vi "Main.vi"(8 "error in":errorcluster, 11 "Caméra UI in":refnum<class "Caméra UI.lvclass">) -> (0 "error out":errorcluster, 3 "Caméra UI out":refnum<class "Caméra UI.lvclass">)   [LabVIEW 2026, in "Caméra UI.lvclass"]
doc: "The <b>Queued Message Handler</b> of the Worker that owns this VI."
uses:
  C:/Program Files/National Instruments/LabVIEW 2026/vi.lib/addons/_Workers/Library/Classes/Worker/Worker.lvclass
  Initialization Data.ctl
  Response Cases.ctl
  <vilib>/addons/_Workers/Library/Classes/Message Queue/Message Queue.lvclass
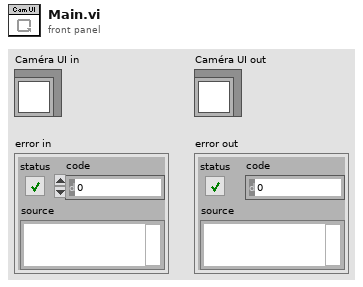
[diagram p1: front panel]
types:
  T1 = typedef "Caméra UI.lvclass/Initialization Data.ctl" = cluster{"Response Cases":T2}
  T2 = typedef "Caméra UI.lvclass/Response Cases.ctl" = cluster{"Placeholder - Can be deleted":string}
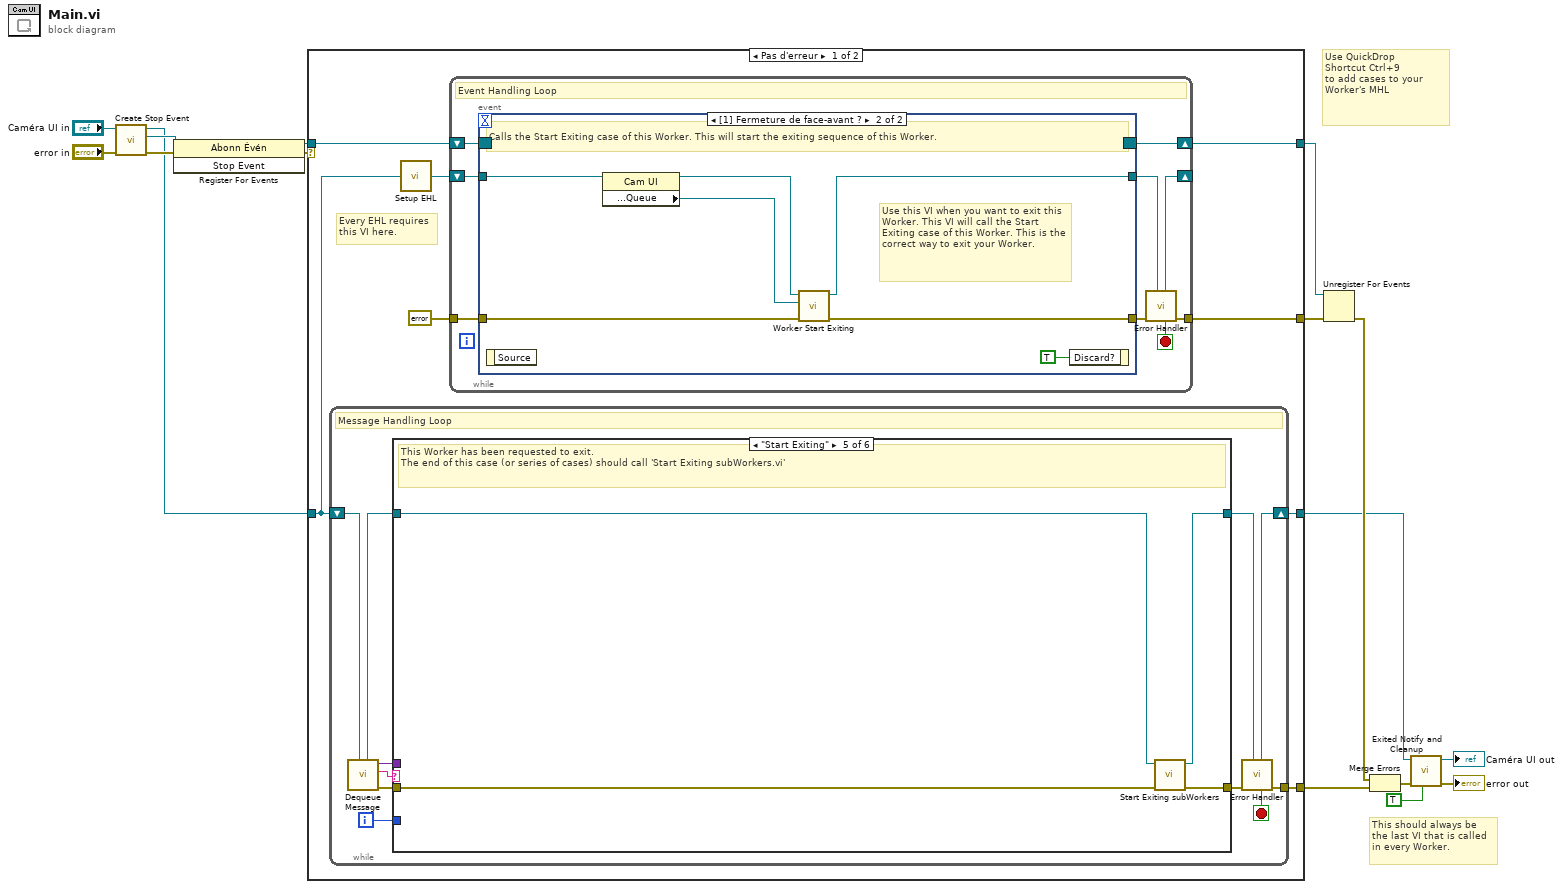
[diagram p0: block diagram]
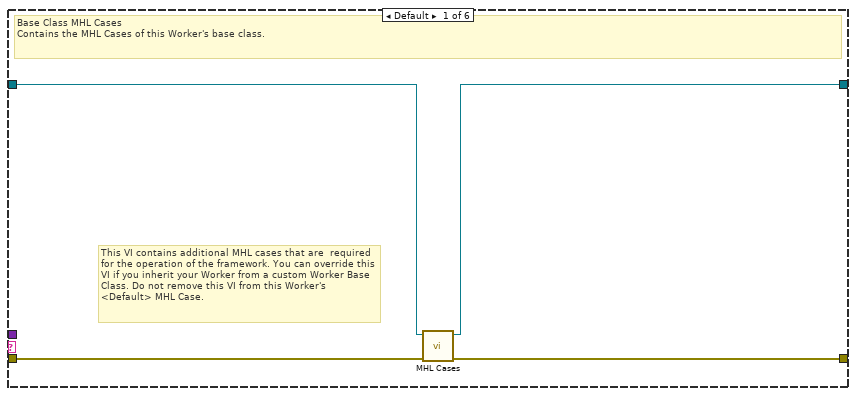
[diagram p2: hidden frame]
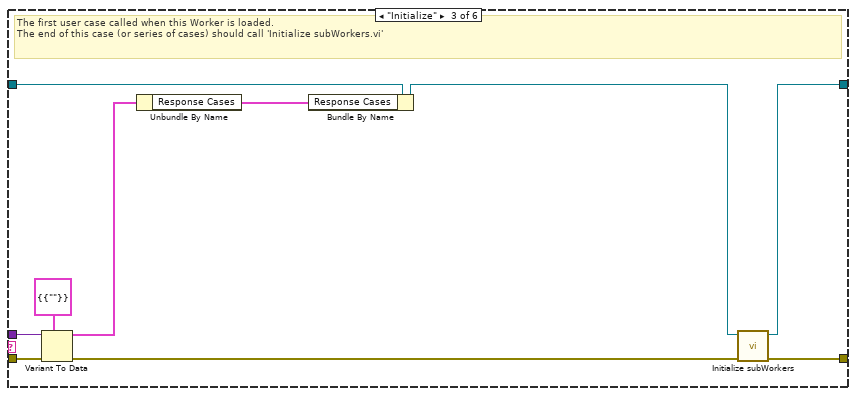
[diagram p4: hidden frame]
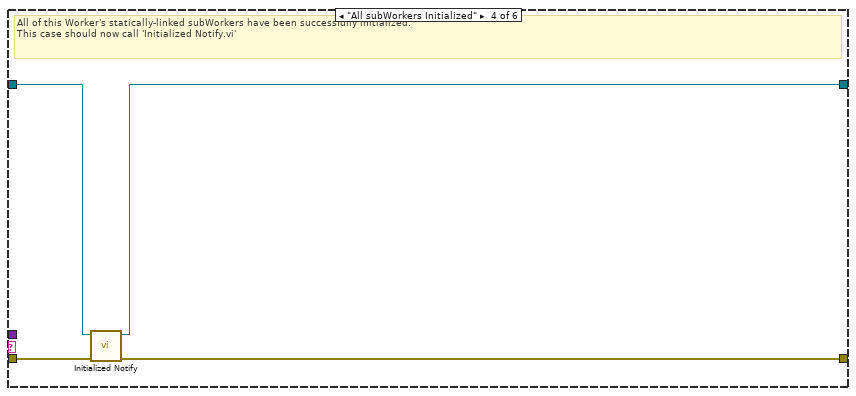
[diagram p5: hidden frame]
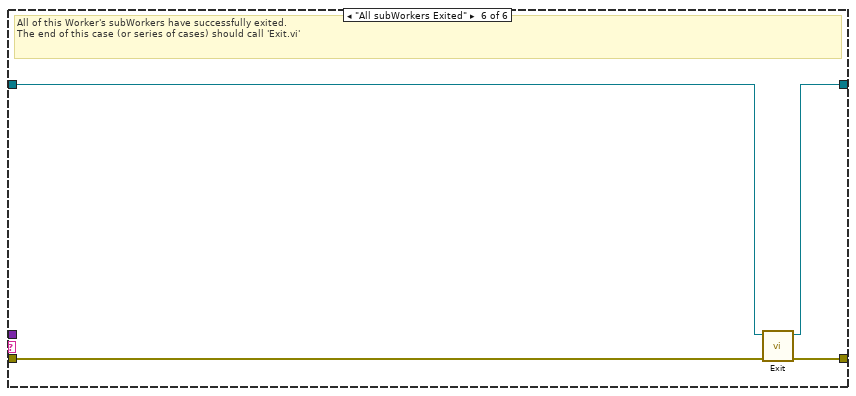
[diagram p6: hidden frame]
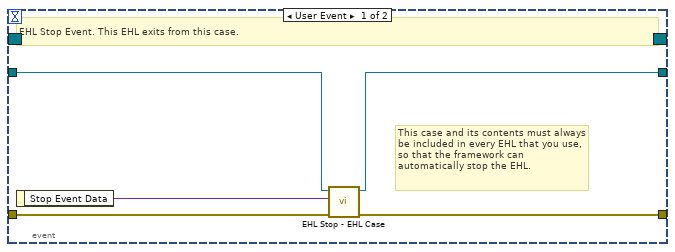
[diagram p7: hidden frame]
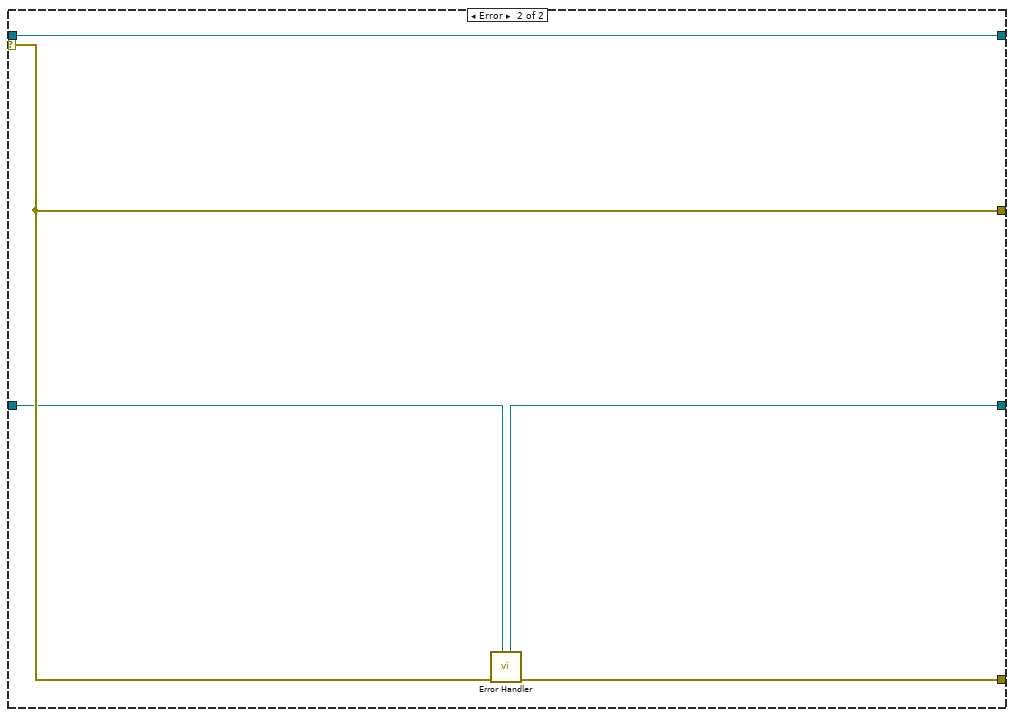
[diagram p8: hidden frame]
diagram:
  # "Use QuickDrop\nShortcut Ctrl+9\nto add cases to your\nWorker's MHL"
  # "This should always be the last VI that is called in every Worker."
  n1 = call-dynamic "Create Stop Event.vi"("error in"="error in", "Worker"="Caméra UI in") -> ("error out"=w11:errorcluster, "Stop Event"=w8:refnum<user-event>, "Worker out"=w5:refnum<class "Caméra UI.lvclass">)  [unwired: 7 in]
  n2 = register-events(error in=w11, w8) -> (reference out=w10:refnum<event-registration>, error out=w2:errorcluster)  [unwired: 1 in]
  n3 = case shown="Pas d'erreur" w2 {
    tunnel: w5 -> [w19 w86]
    tunnel: [w17 w87] -> w9
    tunnel: w10 -> [w24 w88]
    tunnel: [w21 w89] -> w15
    tunnel: [w23 w88] -> w14
    tunnel: [w18 w85] -> w12
    selector: w2 -> [_ w89]
    frame No Error {
      # "Every EHL requires\nthis VI here."
      n4 = while {
        shift-right: [w33] -> w18
        shift-left: w19 -> [w35]
        tunnel: [w34] -> w17
        i -> [w25]
        stop <- w26 stop-if-true
        # "Message Handling Loop"
        n5 = call-dynamic "Dequeue Message.vi"("Worker"=w35) -> ("error out"=w32:errorcluster, "Case out"=w27:string, "Data out"=w28:variant, "Worker out"=w30:refnum<class "Caméra UI.lvclass">)  [unwired: 6 in, 1 out]
        n6 = case "Worker MHL Case Structure (DO NOT CHANGE LABEL NAME)" shown="\"Start Exiting\"" w27 {
          tunnel: w32 -> [w39 w40 w49 w53 w56 w63]
          tunnel: [w38 w40 w51 w52 w59 w62] -> w31
          tunnel: w30 -> [w37 w41 w48 w55 w57 w61]
          tunnel: [w36 w41 w50 w54 w58 w60] -> w29
          tunnel: w28 -> [_ _ w46 _ _ _]
          tunnel: w25 -> [_ _ _ _ _ _]
          frame Default {
            # "This VI contains additional MHL cases that are  required for the operation of the framework. You can override this VI if you inherit your Worker from a custom Worker Base Class. Do not remove this VI from this Worker's <Default> MHL Case."
            # "Base Class MHL Cases\nContains the MHL Cases of this Worker's base class."
            n7 = call-dynamic "MHL Cases.vi"("error in"=w39, "Worker in"=w37) -> ("error out"=w38:errorcluster, "Worker out"=w36:refnum<class "Caméra UI.lvclass">)  [unwired: 8 in]
          }
          frame "------------ FRAMEWORK CASES -----------" {
            # "Start of Workers Framework Cases"
          }
          frame "Initialize" {
            # "The first user case called when this Worker is loaded.\nThe end of this case (or series of cases) should call 'Initialize subWorkers.vi'"
            n8 = Variant To Data(error in=w49, type=T1 {"Response Cases"={"Placeholder - Can be deleted"=""}} ("Initialization Data"), Variant=w46) -> (data=w44:T1, error out=w47:errorcluster)
            n9 = Unbundle By Name(w44) -> ("Response Cases"=w43:T2)
            n10 = Bundle By Name(cluster=w48, "Response Cases"=w43) -> (w45:refnum<class "Caméra UI.lvclass">)
            n11 = call-dynamic "Initialize subWorkers.vi"("error in"=w47, "Worker"=w45) -> ("error out"=w51:errorcluster, "dup Worker out"=w50:refnum<class "Caméra UI.lvclass">)  [unwired: 8 in]
          }
          frame "All subWorkers Initialized" {
            # "All of this Worker's statically-linked subWorkers have been successfully initialized.\nThis case should now call 'Initialized Notify.vi'"
            n12 = call-dynamic "Initialized Notify.vi"("error in"=w53, "Worker"=w55) -> ("error out"=w52:errorcluster, "dup Worker out"=w54:refnum<class "Caméra UI.lvclass">)  [unwired: 8 in]
          }
          frame "Start Exiting" {
            # "This Worker has been requested to exit. \nThe end of this case (or series of cases) should call 'Start Exiting subWorkers.vi'"
            n13 = call-dynamic "Start Exiting subWorkers.vi"("error_in"=w56, "Worker"=w57) -> ("error out"=w59:errorcluster, "dup Worker out"=w58:refnum<class "Caméra UI.lvclass">)  [unwired: 8 in]
          }
          frame "All subWorkers Exited" {
            # "All of this Worker's subWorkers have successfully exited. \nThe end of this case (or series of cases) should call 'Exit.vi'"
            n14 = call-dynamic "Exit.vi"("error_in"=w63, "Worker"=w61) -> ("error out"=w62:errorcluster, "dup Worker out"=w60:refnum<class "Caméra UI.lvclass">)  [unwired: 8 in]
          }
        }
        n15 = call-dynamic "Error Handler.vi"("Worker"=w29, "error_in"=w31) -> ("error out"=w34:errorcluster, "Stop Loop"=w26:bool, "Worker out"=w33:refnum<class "Caméra UI.lvclass">)  [unwired: 7 in]
      }
      n16 = call-dynamic "Setup EHL.vi"("Worker"=w19) -> ("Worker out"=w20:refnum<class "Caméra UI.lvclass">)  [unwired: 14 in]
      n17 = while "Event Handling Loop" {
        shift-right: [w72] -> w23
        shift-left: w24 -> [w71]
        tunnel: [w67] -> w21
        tunnel: errorcluster {"status"=FALSE, "code"=0, "source"=""} ("error constant") -> [w69]
        shift-right: [w65] -> _
        shift-left: w20 -> [w70]
        stop <- w64 stop-if-true
        # "Event Handling Loop"
        n18 = event shown="[1] Fermeture de face-avant ?" {
          selector: w71 -> [_ _]
          dyn-events: [_ _] -> w72
          timeout: _ -> [_ _]
          tunnel: [w76 w83] -> w68
          tunnel: w69 -> [w77 w82]
          tunnel: w70 -> [w75 w81]
          tunnel: [w74 w80] -> w66
          event User Event {
            # "This case and its contents must always be included in every EHL that you use, so that the framework can automatically stop the EHL."
            # "EHL Stop Event. This EHL exits from this case."
            n19 = event-data() -> ("Stop Event Data"=w73:variant)  [unwired: 1 in]
            n20 = call-dynamic "EHL Stop - EHL Case.vi"("error in"=w77, "Stop Event Data"=w73, "Worker"=w75) -> ("error out"=w76:errorcluster, "Worker out"=w74:refnum<class "Caméra UI.lvclass">)  [unwired: 7 in]
          }
          event Panel Close? {
            # "Use this VI when you want to exit this Worker. This VI will call the Start Exiting case of this Worker. This is the correct way to exit your Worker."
            # "Calls the Start Exiting case of this Worker. This will start the exiting sequence of this Worker."
            n21 = event-data() -> ()  [unwired: 1 in, 1 out]
            n22 = property class="Cam UI"(reference=w81) -> (reference out=w79:refnum<class "Caméra UI.lvclass">, "Accessors:Read:Public API:Queue"=w78:refnum<class "Message Queue.lvclass">)  [unwired: 1 in, 1 out]
            n23 = call-dynamic "Worker Start Exiting.vi"("error_in"=w82, "Message Queue"=w78, "Worker"=w79) -> ("error out"=w83:errorcluster, "dup Worker out"=w80:refnum<class "Caméra UI.lvclass">)  [unwired: 7 in]
            n24 = event-data("Discard?"=TRUE) -> ()  [unwired: 1 in, 1 out]
          }
        }
        n25 = call-dynamic "Error Handler.vi"("Worker"=w66, "error_in"=w68) -> ("error out"=w67:errorcluster, "Stop Loop"=w64:bool, "Worker out"=w65:refnum<class "Caméra UI.lvclass">)  [unwired: 7 in]
      }
    }
    frame Error {
      n26 = call-dynamic "Error Handler.vi"("Worker"=w86, "error_in"=w89) -> ("error out"=w87:errorcluster, "Worker out"=w85:refnum<class "Caméra UI.lvclass">)  [unwired: 7 in, 1 out]
    }
  }
  n27 = Unregister For Events(event registration refnum=w14, error in=w15) -> (error out=w16:errorcluster)
  n28 = Merge Errors(w16, w9) -> (w13:errorcluster)
  n29 = call-dynamic "Exited Notify and Cleanup.vi"("Close FP on Exit? (T)"=TRUE, "error_in"=w13, "Worker"=w12) -> ("error out"=→"error out":errorcluster, "dup Worker out"=→"Caméra UI out":refnum<class "Caméra UI.lvclass">)  [unwired: 7 in]
